vi "FRIC_navX_Internal_ProcessingLoop_UpdateAE.vi"(0 "Device Number":T1) -> (1 "Board Information":T12 {"Board"."Hardware Revision" items=["navX-MXP"=33, "navX-Micro"=40]; "Omnimount Config" items=["DEFAULT", "X_UP", "X_DOWN", "Y_UP", "Y_DOWN", "Z_UP", "Z_DOWN"]}, 2 "MPUTemp":dbl, 3 "Displacement":T13, 4 "Linear Acceleration":T9, 6 "Offsets":T8, 8 "Quaternion":T6, 10 "YRPHfH":T2, 12 "Raw Values (out)":T7, 13 "Status":T5 {"OP Status" items=["INITIALIZING", "SELFTEST_IN_PROGRESS", "ERROR", "IMU_AUTOCAL_IN_PROGRESS", "NORMAL"]; "Calibration Status" items=["IMU_CAL_STATE_MASK"=3, "IMU_CAL_STATE_INPROGRESS"=0, "IMU_CAL_STATE_ACCUMULATE"=1, "IMU_CAL_STATE_COMPLETE"=2]}, 14 "Timestamp":u32)   [LabVIEW 2015]
uses:
  _TypeDefs/Flags/Z900_navX_Flags_HardwareRevTypeDef.ctl
  _TypeDefs/Flags/Z900_navX_Flags_OmnimountConfigTypeDef.ctl
  _TypeDefs/Flags/Z900_navX_Flags_OpStatusTypeDef.ctl
  _TypeDefs/Flags/Z900_navX_Flags_CalibrationStatusTypeDef.ctl
  _TypeDefs/FRIC_navX_DeviceNumbersTypeDef.ctl
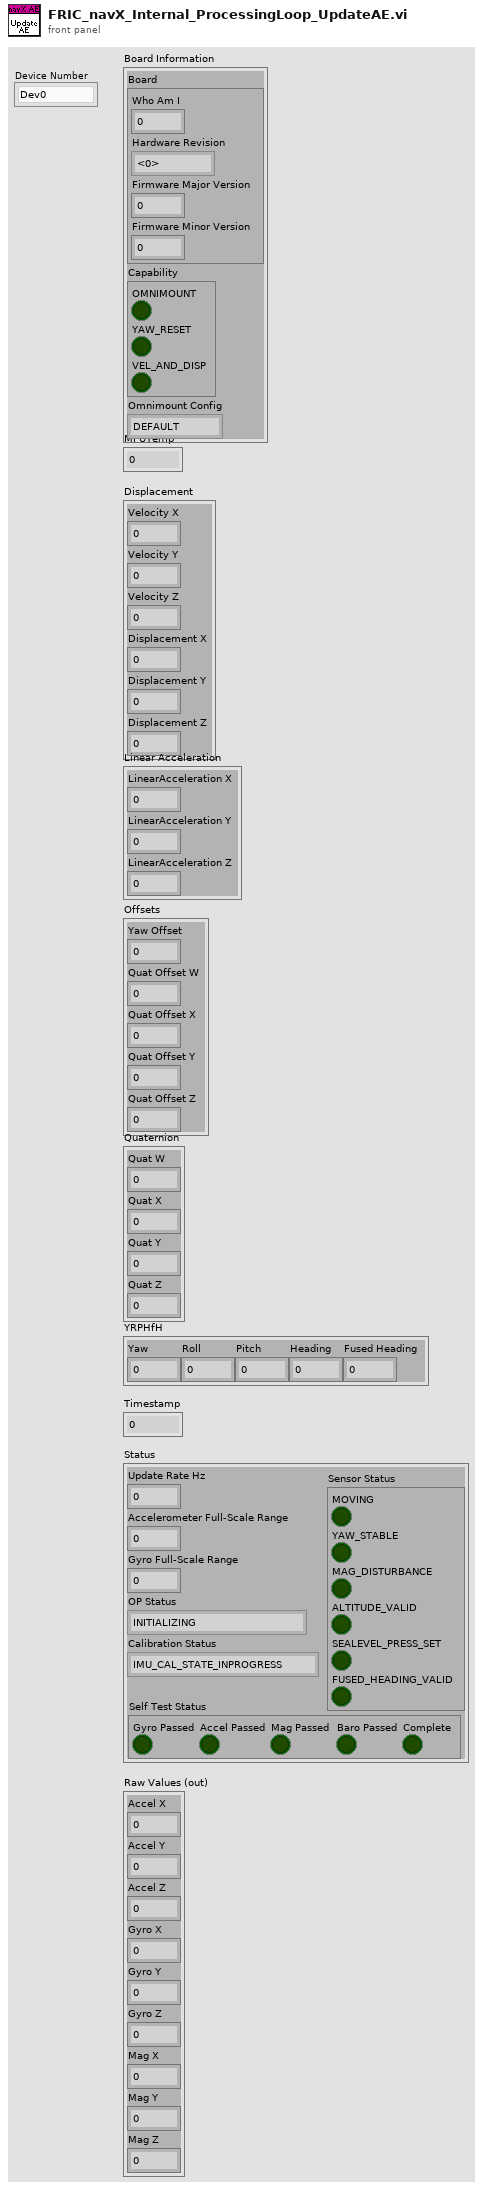
[diagram p1: front panel]
types:
  T1 = typedef "FRIC_navX_DeviceNumbersTypeDef.ctl" = enum16{"Dev0", "Dev1", "Dev2", "Dev3", "Dev4", "Dev5", "Dev6", "Dev7", "Dev8", "Dev9", "Dev10"}
  T2 = cluster{"Yaw":dbl, "Roll":dbl, "Pitch":dbl, "Heading":dbl, "Fused Heading":dbl}
  T3 = typedef "Z900_navX_Flags_OpStatusTypeDef.ctl" = u8
  T4 = typedef "Z900_navX_Flags_CalibrationStatusTypeDef.ctl" = u8
  T5 = cluster{"Update Rate Hz":u8, "Accelerometer Full-Scale Range":u8, "Gyro Full-Scale Range":u16, "OP Status":T3, "Calibration Status":T4, "Sensor Status":cluster{"MOVING":bool, "YAW_STABLE":bool, "MAG_DISTURBANCE":bool, "ALTITUDE_VALID":bool, "SEALEVEL_PRESS_SET":bool, "FUSED_HEADING_VALID":bool}, "Self Test Status":cluster{"Gyro Passed":bool, "Accel Passed":bool, "Mag Passed":bool, "Baro Passed":bool, "Complete":bool}}
  T6 = cluster{"Quat W":dbl, "Quat X":dbl, "Quat Y":dbl, "Quat Z":dbl}
  T7 = cluster{"Accel X":dbl, "Accel Y":dbl, "Accel Z":dbl, "Gyro X":dbl, "Gyro Y":dbl, "Gyro Z":dbl, "Mag X":dbl, "Mag Y":dbl, "Mag Z":dbl}
  T8 = cluster{"Yaw Offset":dbl, "Quat Offset W":dbl, "Quat Offset X":dbl, "Quat Offset Y":dbl, "Quat Offset Z":dbl}
  T9 = cluster{"LinearAcceleration X":dbl, "LinearAcceleration Y":dbl, "LinearAcceleration Z":dbl}
  T10 = typedef "Z900_navX_Flags_HardwareRevTypeDef.ctl" = u8
  T11 = typedef "Z900_navX_Flags_OmnimountConfigTypeDef.ctl" = u8
  T12 = cluster{"Board":cluster{"Who Am I":u8, "Hardware Revision":T10, "Firmware Major Version":u8, "Firmware Minor Version":u8}, "Capability":cluster{"OMNIMOUNT":bool, "YAW_RESET":bool, "VEL_AND_DISP":bool}, "Omnimount Config":T11}
  T13 = cluster{"Velocity X":dbl, "Velocity Y":dbl, "Velocity Z":dbl, "Displacement X":dbl, "Displacement Y":dbl, "Displacement Z":dbl}
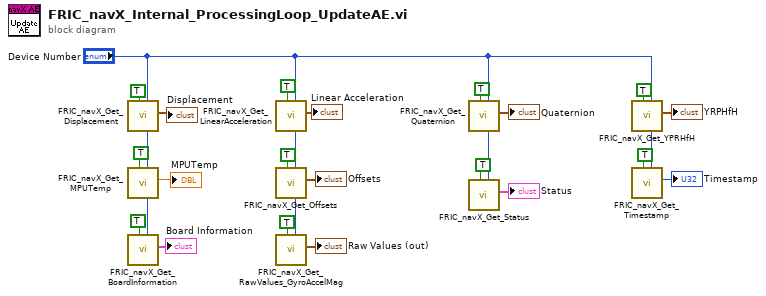
[diagram p0: block diagram]
diagram:
  n1 = call "FRIC_navX_Get_Displacement.vi"("Device Number"="Device Number", "Update"=TRUE) -> ("Displacement"=→"Displacement":T13)  [unwired: 9 in]
  n2 = call "FRIC_navX_Get_MPUTemp.vi"("Device Number"="Device Number", "Update"=TRUE) -> ("MPUTemp"=→"MPUTemp":dbl)  [unwired: 9 in]
  n3 = call "FRIC_navX_Get_BoardInformation.vi"("Device Number"="Device Number", "Update"=TRUE) -> ("Board Information"=→"Board Information":T12)  [unwired: 9 in]
  n4 = call "FRIC_navX_Get_LinearAcceleration.vi"("Device Number"="Device Number", "Update"=TRUE) -> ("Linear Acceleration"=→"Linear Acceleration":T9)  [unwired: 9 in]
  n5 = call "FRIC_navX_Get_Offsets.vi"("Device Number"="Device Number", "Update"=TRUE) -> ("Offsets"=→"Offsets":T8)  [unwired: 9 in]
  n6 = call "FRIC_navX_Get_RawValues_GyroAccelMag.vi"("Device Number"="Device Number", "Update"=TRUE) -> ("Raw Values (out)"=→"Raw Values (out)":T7)  [unwired: 9 in]
  n7 = call "FRIC_navX_Get_Quaternion.vi"("Device Number"="Device Number", "Update"=TRUE) -> ("Quaternion"=→"Quaternion":T6)  [unwired: 9 in]
  n8 = call "FRIC_navX_Get_Status.vi"("Device Number"="Device Number", "Update"=TRUE) -> ("Status"=→"Status":T5)  [unwired: 9 in]
  n9 = call "FRIC_navX_Get_YPRHfH.vi"("Device Number"="Device Number", "Update"=TRUE) -> ("YRPHfH"=→"YRPHfH":T2)  [unwired: 9 in]
  n10 = call "FRIC_navX_Get_Timestamp.vi"("Device Number"="Device Number", "Update"=TRUE) -> ("Timestamp"=→"Timestamp":u32)  [unwired: 9 in]
